vi "Configure Load Timer.vi"(8 "error in (no error)":errorcluster, 9 "Timer Value":u32 max=60000, 10 "Enable Load Timer":bool, 11 "VISA resource name":refnum<visa-resource-name>) -> (0 "error out":errorcluster, 3 "VISA resource name out":refnum<visa-resource-name>)   [LabVIEW 2015, in "IT8900A-E.lvlib"]
doc: "These commands enable or disable all electronic load timers.If the energy electronic load timer is enabled, its value is set."
uses:
  <instrlib>/IT8900/IT8900A-E.lvlib
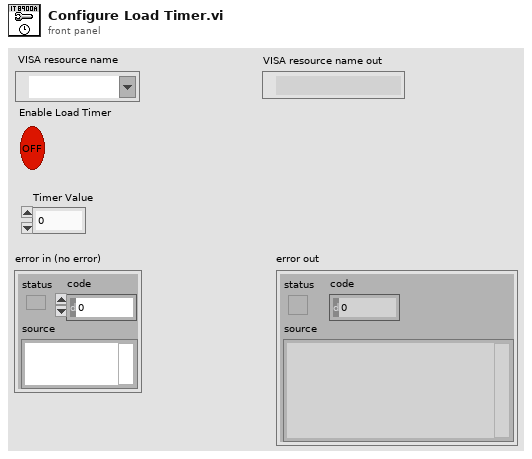
[diagram p1: front panel]
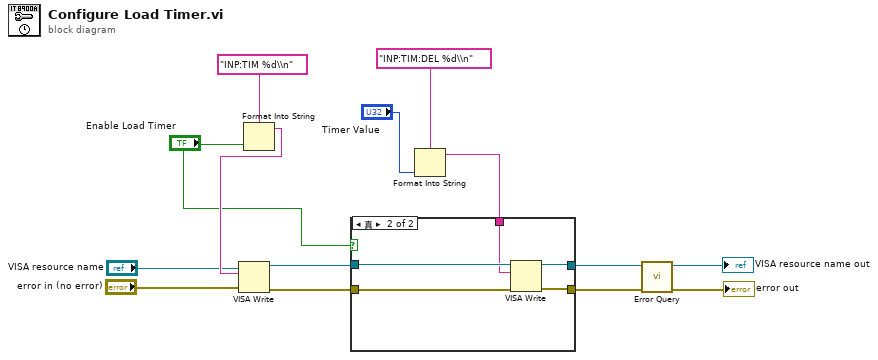
[diagram p0: block diagram]
diagram:
  n1 = Format Into String(format string="INP:TIM %d\\n", "Enable Load Timer") -> (resulting string=w13:string)  [unwired: 2 in, 1 out]
  n2 = VISA Write(VISA resource name="VISA resource name", write buffer=w13, error in (no error)="error in (no error)") -> (VISA resource name out=w3:refnum<visa-resource-name>, error out=w2:errorcluster)  [unwired: 1 out]
  n3 = Format Into String(format string="INP:TIM:DEL %d\\n", "Timer Value") -> (resulting string=w1:string)  [unwired: 2 in, 1 out]
  n4 = case shown="真" "Enable Load Timer" {
    tunnel: [w16 w21] -> w6
    tunnel: [w15 w20] -> w5
    tunnel: w3 -> [w16 w19]
    tunnel: w2 -> [w15 w18]
    tunnel: w1 -> [_ w17]
    frame False {
    }
    frame True {
      n5 = VISA Write(VISA resource name=w19, write buffer=w17, error in (no error)=w18) -> (VISA resource name out=w21:refnum<visa-resource-name>, error out=w20:errorcluster)  [unwired: 1 out]
    }
  }
  n6 = call <instrlib>:"Error Query.vi"("error in (no error)"=w5, "VISA resource name"=w6) -> ("error out"=→"error out":errorcluster, "VISA resource name out"=→"VISA resource name out":refnum<visa-resource-name>)  [unwired: 6 in, 2 out]
